vi "Loop Practice.vi"() -> ()   [LabVIEW 2016]
uses:
  <vilib>/express/express arith-compare/Formula/XNode/ExpressFormulaBlockNode.xnode
panel:
  out "n":dbl
  out "InvSum":dbl
  out "Total":dbl
  in  "n":dbl
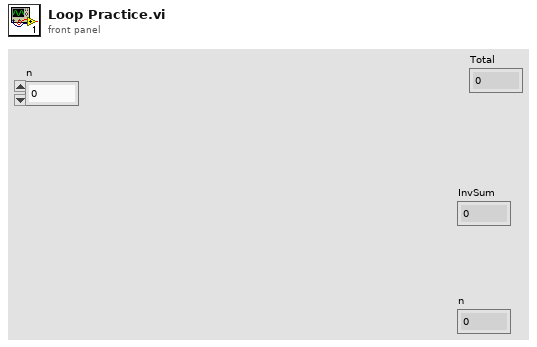
[diagram p1: front panel]
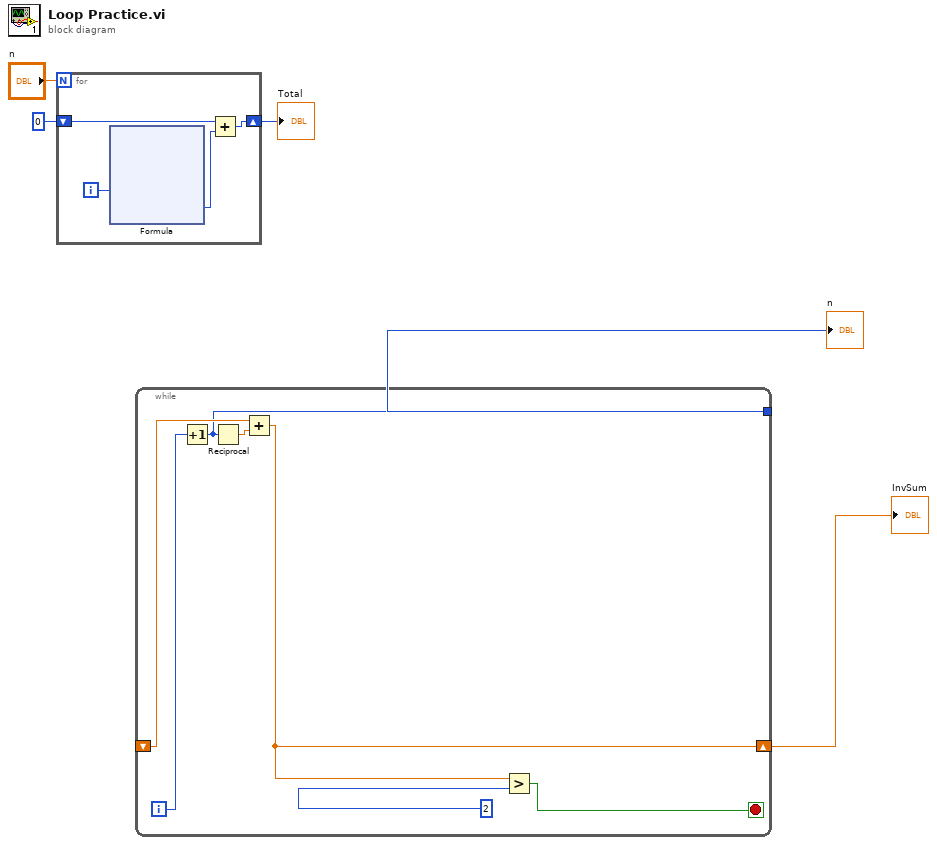
[diagram p0: block diagram]
diagram:
  n1 = for {
    N: "n" -> [_]
    shift-right: [w8] -> w5
    shift-left: 0 -> [w6]
    i -> [w9]
    n2 = xnode "Formula"("i"=w9) -> ("Result"=w7:i32)  [unwired: 1 in, 1 out]
    n3 = Add(x=w6, y=w7) -> (x+y=w8:i32)
  }
  "Total" <- w5
  n4 = while {
    shift-right: [w21] -> w2
    shift-left: _ -> [w20]
    tunnel: [w18] -> w1
    i -> [w19]
    stop <- w22 stop-if-true
    n5 = Increment(x=w19) -> (x+1=w18:i32)
    n6 = Reciprocal(x=w18) -> (1/x=w24:dbl)
    n7 = Add(x=w20, y=w24) -> (x+y=w21:dbl)
    n8 = Greater?(x=w21, y=2) -> (0:w22:bool)
  }
  "InvSum" <- w2
  "n" <- w1
